vi "Pockels Cal-Condit mismatch dialogue.vi"(6 "New cal section to be added":bool, 9 "Function":T2(ring)=enum."Conditions mismatch", 11 "Cal conditions":T3) -> (1 "Button pressed":T1, 3 "Continue?":bool)   [LabVIEW 2013]
uses:
  Typedefs/Pockels cal conditions cluster.ctl
  Typedefs/Button Pressed.ctl
  Globals/gl_Calibration globals.vi
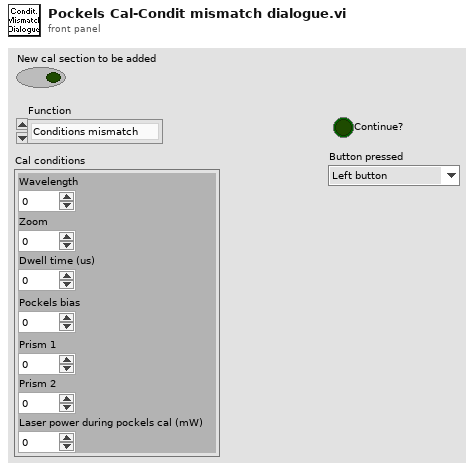
[diagram p1: front panel]
types:
  T1 = typedef "Button Pressed.ctl" = enum16{"Left button", "Middle button", "Right button"}
  T2 = enum16{"Continue anyway", "Conditions match", "Conditions mismatch"}
  T3 = typedef "Pockels cal conditions cluster.ctl" = cluster{"Wavelength":u16, "Zoom":u8, "Dwell time (us)":dbl, "Pockels bias":i16, "Prism 1":u16, "Prism 2":u16, "Laser power during pockels cal (mW)":u16}
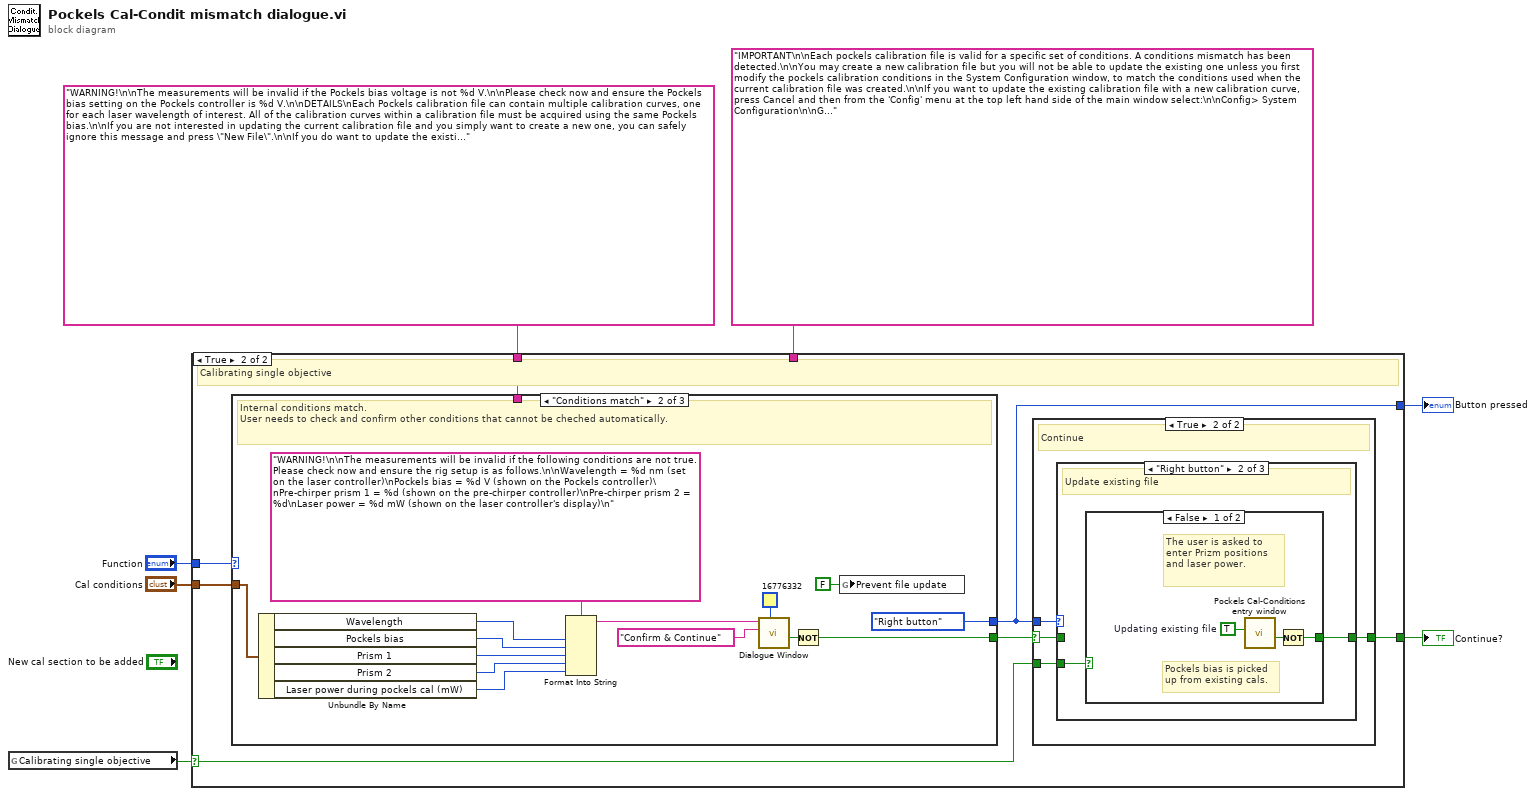
[diagram p0: block diagram]
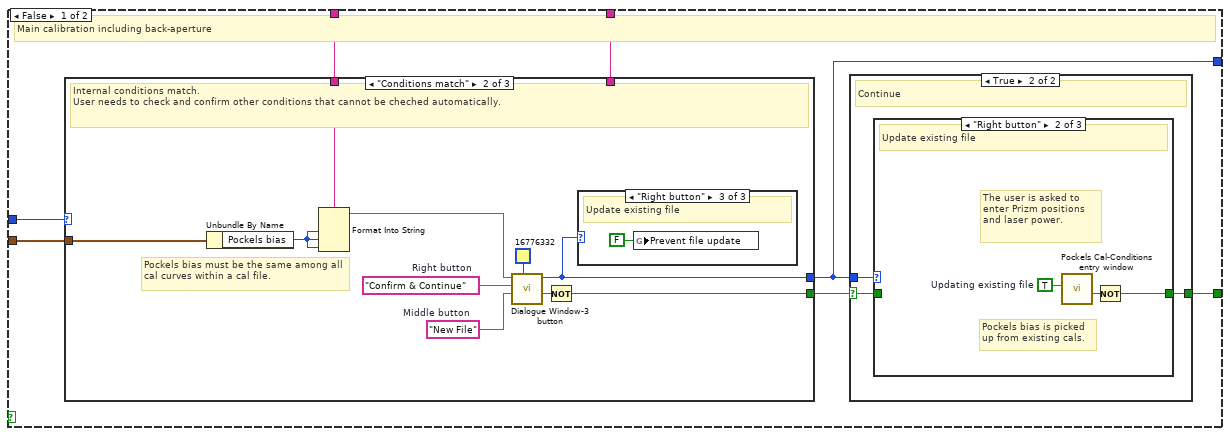
[diagram p2: hidden frame]
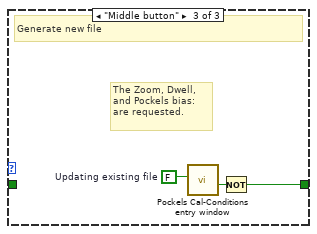
[diagram p5: hidden frame]
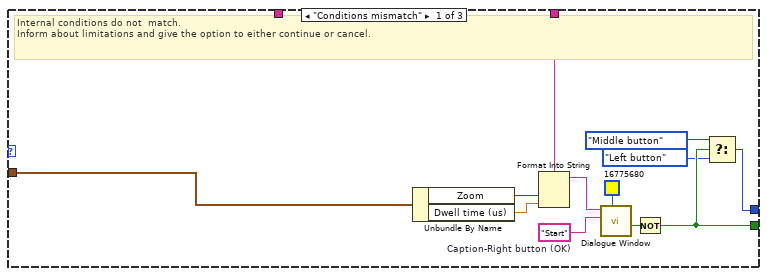
[diagram p6: hidden frame]
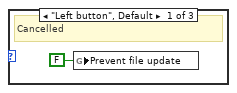
[diagram p7: hidden frame]
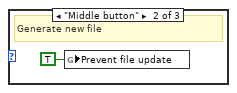
[diagram p8: hidden frame]
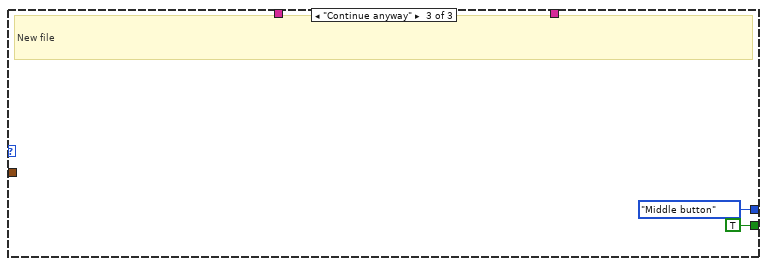
[diagram p9: hidden frame]
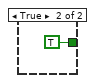
[diagram p12: hidden frame]
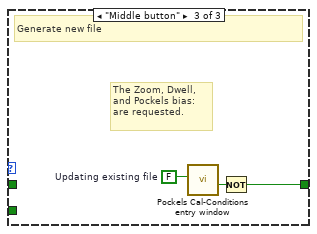
[diagram p13: hidden frame]
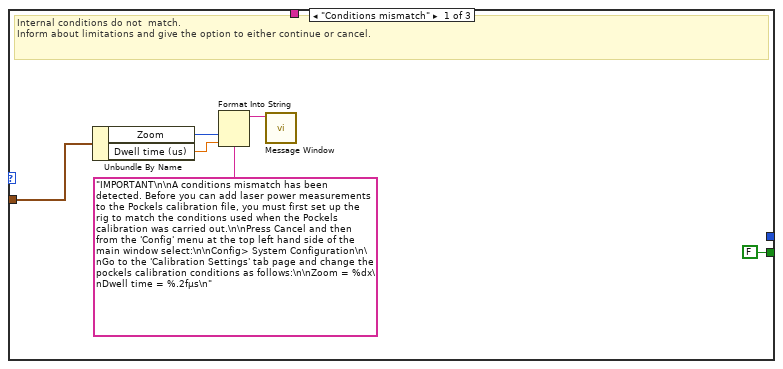
[diagram p14: hidden frame]
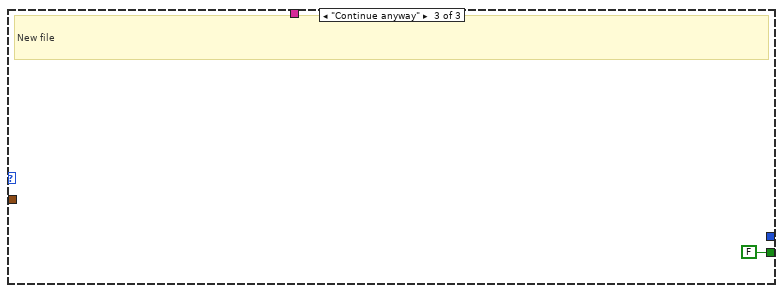
[diagram p15: hidden frame]
diagram:
  n1 = global read "gl_Calibration globals.vi" "Calibrating single objective"() -> (w1:bool)
  n2 = case shown="True" w1 {
    selector: w1 -> [_ w53]
    tunnel: "Function" -> [w14 w59]
    tunnel: "IMPORTANT\n\nEach pockels calibration file is valid for a specific set of conditions. A conditions mismatch has been detected.\n\nYou may create a new calibration file but you will not be able to update the existing one unless you first modify the pockels calibration conditions in the System Configuration window, to match the conditions used when the current calibration file was created.\n\nIf you want to update the existing calibration file with a new calibration curve, press Cancel and then from the 'Config' menu at the top left hand side of the main window select:\n\nConfig> System Configuration\n\nGo to the 'Calibration Settings' tab page and change the pockels calibration conditions as follows:\n\nZoom = %dx\nDwell time = %.2fµs\n\nIf you are not interested in updating the existing calibration file and you simply want to create a new one, you can safely ignore this message and press \"Start\".\n" ("Message string") -> [w13 _]
    tunnel: "Cal conditions" -> [w12 w58]
    tunnel: [w10 w56] -> w4
    tunnel: [w9 w55] -> w3
    tunnel: "WARNING!\n\nThe measurements will be invalid if the Pockels bias voltage is not %d V.\n\nPlease check now and ensure the Pockels bias setting on the Pockels controller is %d V.\n\nDETAILS\nEach Pockels calibration file can contain multiple calibration curves, one for each laser wavelength of interest. All of the calibration curves within a calibration file must be acquired using the same Pockels bias.\n\nIf you are not interested in updating the current calibration file and you simply want to create a new one, you can safely ignore this message and press \"New File\".\n\nIf you do want to update the existing calibration file with a new calibration curve, please confirm the Pockels bias voltage is %d and press \"Confirm & Continue\".\n" ("Message string") -> [w8 w54]
    frame False {
      # "Main calibration including back-aperture"
      n3 = case shown="\"Conditions match\"" w14 {
        tunnel: [w28 w45 TRUE] -> w11
        tunnel: w13 -> [w31 _ _]
        tunnel: w12 -> [w30 w43 _]
        tunnel: [w29 w40 Button_Pressed."Middle button" ("Button pressed")] -> w10
        tunnel: w8 -> [_ w39 _]
        frame "Conditions mismatch" {
          w35 = "Start"  # Caption-Right button (OK)
          # "Internal conditions do not  match.\nInform about limitations and give the option to either continue or cancel."
          n4 = Unbundle By Name(w30) -> ("Zoom"=w34:u8, "Dwell time (us)"=w33:dbl)
          n5 = Format Into String(format string=w31, w34, w33) -> (resulting string=w32:string)  [unwired: 2 in, 1 out]
          n6 = call "Dialogue Window.vi"("Colour"=u32 16775680, "Caption-Right button (OK)"=w35, "Message string"=w32) -> ("Cancelled (Left button pressed)"=w36:bool)  [unwired: 6 in, 2 out]
          n7 = Not(x=w36) -> (.not. x?=w28:bool)
          n8 = Select(t=Button_Pressed."Middle button" ("Button pressed"), s=w28, f=Button_Pressed."Left button" ("Button pressed")) -> (s? t:f=w29:T1)
        }
        frame "Conditions match" {
          w41 = "New File"  # Middle button
          w42 = "Confirm & Continue"  # Right button
          # "Pockels bias must be the same among all cal curves within a cal file."
          # "Internal conditions match.\nUser needs to check and confirm other conditions that cannot be cheched automatically."
          n9 = Unbundle By Name(w43) -> ("Pockels bias"=w38:i16)
          n10 = Format Into String(format string=w39, w38, w38, w38) -> (resulting string=w44:string)  [unwired: 2 in, 1 out]
          n11 = call "Dialogue Window-3 button.vi"("Colour"=u32 16776332, "Caption-Middle button"=w41, "Caption-Right button (OK)"=w42, "Message string"=w44) -> ("Cancelled (Left button pressed)"=w46:bool, "Button pressed"=w40:T1)  [unwired: 5 in, 1 out]
          n12 = Not(x=w46) -> (.not. x?=w45:bool)
          n13 = case shown="\"Right button\"" w40 {
            frame "Left button", Default {
              # "Cancelled"
              n14 = global write "gl_Calibration globals.vi" "Prevent file update"(FALSE ("Prevent file update")) -> ()
            }
            frame "Middle button" {
              # "Generate new file"
              n15 = global write "gl_Calibration globals.vi" "Prevent file update"(TRUE ("Prevent file update")) -> ()
            }
            frame "Right button" {
              # "Update existing file"
              n16 = global write "gl_Calibration globals.vi" "Prevent file update"(FALSE ("Prevent file update")) -> ()
            }
          }
        }
        frame "Continue anyway" {
          # "New file"
        }
      }
      n17 = case shown="True" w11 {
        selector: w11 -> [w15 w16]
        tunnel: w10 -> [_ w18]
        tunnel: [w15 w17] -> w9
        frame False {
          # "Cancelled"
        }
        frame True {
          # "Continue"
          n18 = case shown="\"Right button\"" w18 {
            tunnel: [w19 w22 w24] -> w17
            tunnel: w16 -> [w19 _ _]
            frame "Left button", Default {
              # "Cancelled"
            }
            frame "Right button" {
              w20 = TRUE  # Updating existing file
              # "Pockels bias is picked\nup from existing cals."
              # "The user is asked to enter Prizm positions and laser power."
              # "Update existing file"
              n19 = call "Pockels Cal-Conditions entry window.vi"("Update existing file"=w20) -> ("Cancelled (Left button pressed)"=w21:bool)  [unwired: 9 in, 1 out]
              n20 = Not(x=w21) -> (.not. x?=w22:bool)
            }
            frame "Middle button" {
              w23 = FALSE  # Updating existing file
              # "The Zoom, Dwell, and Pockels bias: are requested."
              # "Generate new file"
              n21 = call "Pockels Cal-Conditions entry window.vi"("Update existing file"=w23) -> ("Cancelled (Left button pressed)"=w25:bool)  [unwired: 9 in, 1 out]
              n22 = Not(x=w25) -> (.not. x?=w24:bool)
            }
          }
        }
      }
    }
    frame True {
      # "Calibrating single objective"
      n23 = case shown="\"Conditions match\"" w59 {
        tunnel: [FALSE w90 FALSE] -> w57
        tunnel: w58 -> [w78 w94 _]
        tunnel: [_ Button_Pressed."Right button" ("Button pressed") _] -> w56
        tunnel: w54 -> [_ _ _]
        frame "Conditions mismatch" {
          # "Internal conditions do not  match.\nInform about limitations and give the option to either continue or cancel."
          n24 = Unbundle By Name(w78) -> ("Zoom"=w80:u8, "Dwell time (us)"=w79:dbl)
          n25 = Format Into String(format string="IMPORTANT\n\nA conditions mismatch has been detected. Before you can add laser power measurements to the Pockels calibration file, you must first set up the rig to match the conditions used when the Pockels calibration was carried out.\n\nPress Cancel and then from the 'Config' menu at the top left hand side of the main window select:\n\nConfig> System Configuration\n\nGo to the 'Calibration Settings' tab page and change the pockels calibration conditions as follows:\n\nZoom = %dx\nDwell time = %.2fµs\n" ("Message string"), w80, w79) -> (resulting string=w75:string)  [unwired: 2 in, 1 out]
          n26 = call "Message Window.vi"("Message string"=w75) -> ()  [unwired: 10 in, 1 out]
        }
        frame "Conditions match" {
          # "Internal conditions match.\nUser needs to check and confirm other conditions that cannot be cheched automatically."
          n27 = Unbundle By Name(w94) -> ("Wavelength"=w81:u16, "Pockels bias"=w82:i16, "Prism 1"=w85:u16, "Prism 2"=w84:u16, "Laser power during pockels cal (mW)"=w83:u16)
          n28 = Format Into String(format string="WARNING!\n\nThe measurements will be invalid if the following conditions are not true. Please check now and ensure the rig setup is as follows.\n\nWavelength = %d nm (set on the laser controller)\nPockels bias = %d V (shown on the Pockels controller)\nPre-chirper prism 1 = %d (shown on the pre-chirper controller)\nPre-chirper prism 2 = %d\nLaser power = %d mW (shown on the laser controller's display)\n" ("Message string"), w81, w82, w85, w84, w83) -> (resulting string=w92:string)  [unwired: 2 in, 1 out]
          n29 = call "Dialogue Window.vi"("Colour"=u32 16776332, "Caption-Right button (OK)"="Confirm & Continue", "Message string"=w92) -> ("Cancelled (Left button pressed)"=w91:bool)  [unwired: 6 in, 2 out]
          n30 = Not(x=w91) -> (.not. x?=w90:bool)
          n31 = global write "gl_Calibration globals.vi" "Prevent file update"(FALSE ("Prevent file update")) -> ()
        }
        frame "Continue anyway" {
          # "New file"
        }
      }
      n32 = case shown="True" w57 {
        selector: w57 -> [w60 w62]
        tunnel: w56 -> [_ w64]
        tunnel: [w60 w63] -> w55
        tunnel: w53 -> [_ w61]
        frame False {
          # "Cancelled"
        }
        frame True {
          # "Continue"
          n33 = case shown="\"Right button\"" w64 {
            tunnel: [w65 w67 w73] -> w63
            tunnel: w62 -> [w65 _ _]
            tunnel: w61 -> [_ w66 _]
            frame "Left button", Default {
              # "Cancelled"
            }
            frame "Right button" {
              # "Update existing file"
              n34 = case shown="False" w66 {
                tunnel: [w70 TRUE] -> w67
                frame False {
                  w68 = TRUE  # Updating existing file
                  # "Pockels bias is picked\nup from existing cals."
                  # "The user is asked to enter Prizm positions and laser power."
                  n35 = call "Pockels Cal-Conditions entry window.vi"("Update existing file"=w68) -> ("Cancelled (Left button pressed)"=w69:bool)  [unwired: 9 in, 1 out]
                  n36 = Not(x=w69) -> (.not. x?=w70:bool)
                }
                frame True {
                }
              }
            }
            frame "Middle button" {
              w72 = FALSE  # Updating existing file
              # "The Zoom, Dwell, and Pockels bias: are requested."
              # "Generate new file"
              n37 = call "Pockels Cal-Conditions entry window.vi"("Update existing file"=w72) -> ("Cancelled (Left button pressed)"=w74:bool)  [unwired: 9 in, 1 out]
              n38 = Not(x=w74) -> (.not. x?=w73:bool)
            }
          }
        }
      }
    }
  }
  "Continue?" <- w3
  "Button pressed" <- w4
